vi "Initialize Sweep Waveform.vi"(8 "error in (no error)":errorcluster, 11 "Generator in":refnum<class "Generator.lvclass">) -> (0 "error out":errorcluster, 2 "Waveforms":waveform(dbl)[](array[waveform]), 3 "Generator out":refnum<class "Generator.lvclass">)   [LabVIEW 2019, in "Generator.lvclass"]
uses:
  Generator.lvclass
  Generator.lvclass/Generator.ctl
  <vilib>/Utility/error.llb/Error Cluster From Error Code.vi
  <vilib>/ErrorRing/Error Ring.xnode
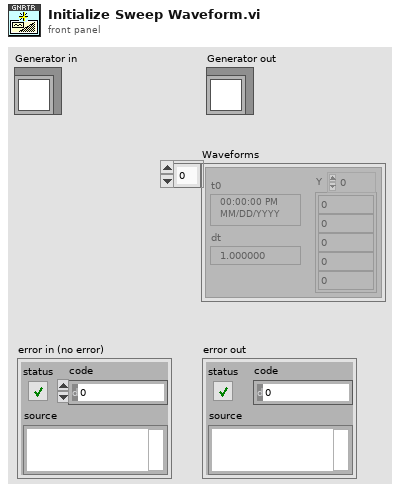
[diagram p1: front panel]
types:
  T1 = typedef "Generator.lvclass/AO.Channel--Cluster--Array.ctl" = T2[]
  T2 = typedef "Generator.lvclass/AO.Channel--Cluster.ctl" = cluster{"Enable?":bool, "Channel":i32, "Amplitude":dbl, "Offset":dbl, "Frequency":dbl, "Phase":dbl, "Function":T3, "Sweeping?":bool, "Limit AC?":bool, "Limit DC?":bool, "Duty Cycle?":bool, "Duty Cycle":dbl}
  T3 = typedef "Generator.lvclass/AO.Channel.Function--Enum.ctl" = enum16{"sine", "square", "triangle", "saw"}
  T4 = typedef "Generator.lvclass/Sweep.Channel--Cluster--Array.ctl" = T5[]
  T5 = typedef "Generator.lvclass/Sweep.Channel--Cluster.ctl" = cluster{"Enable?":bool, "Channel":u16, "Start":dbl, "End":dbl, "Pattern":T6, "Table":dbl[]}
  T6 = typedef "Generator.lvclass/Sweep.Pattern--Enum.ctl" = enum16{"Ramp /", "Ramp /\\", "Smooth Ramp _/", "Smooth Ramp _/\\_", "Table"}
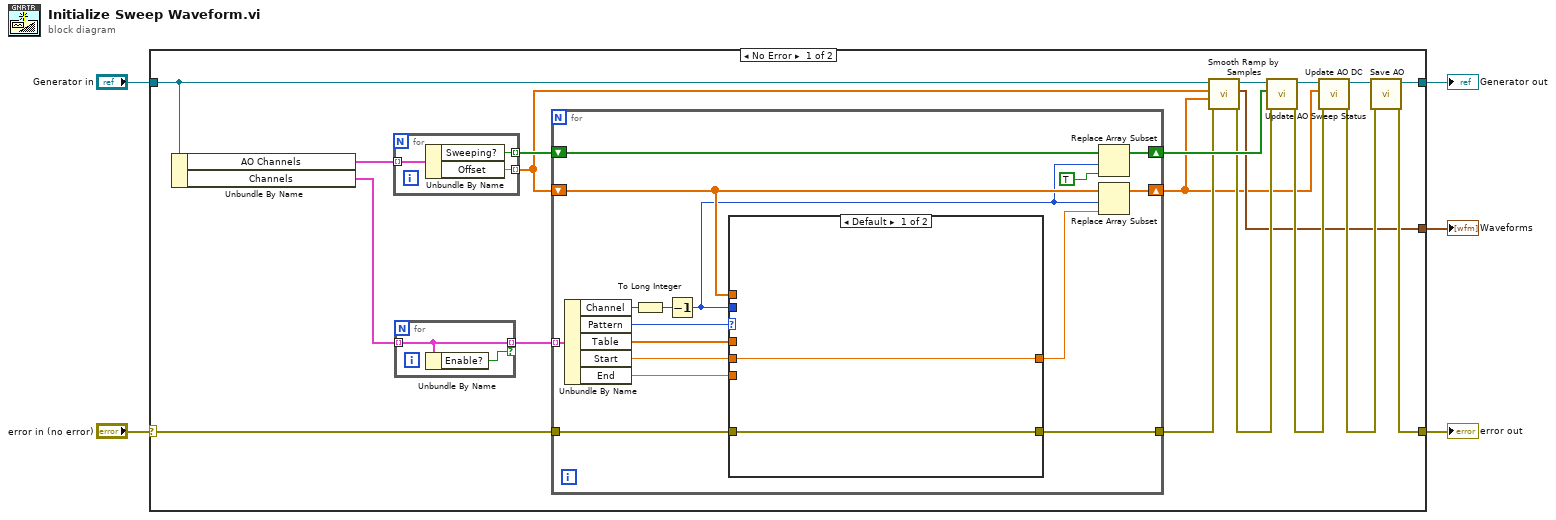
[diagram p0: block diagram]
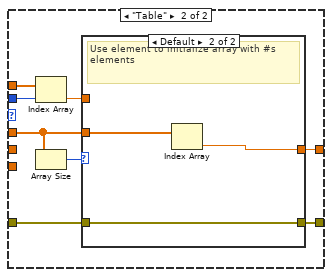
[diagram p2: hidden frame]
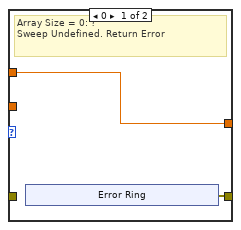
[diagram p3: hidden frame]
diagram:
  n1 = case shown="No Error" "error in (no error)" {
    selector: "error in (no error)" -> [w11 w67]
    tunnel: "Generator in" -> [w12 w66]
    tunnel: [w15 w67] -> w2
    tunnel: [w14 w66] -> w1
    tunnel: [w7 _] -> w3
    frame No Error {
      n2 = Unbundle By Name(w12) -> ("AO Channels"=w22:T1, "Channels"=w21:T4)
      n3 = for {
        tunnel: [w65] -> w8 mode=indexing
        tunnel: [w64] -> w23 mode=indexing
        tunnel: w22 -> [w63] mode=indexing
        n4 = Unbundle By Name(w63) -> ("Sweeping?"=w64:bool, "Offset"=w65:dbl)
      }
      n5 = for {
        tunnel: w21 -> [w62] mode=indexing
        tunnel: [w62] -> w24 mode=indexing if=w61
        n6 = Unbundle By Name(w62) -> ("Enable?"=w61:bool)
      }
      n7 = for {
        tunnel: w11 -> [w40]
        tunnel: w24 -> [w35] mode=indexing
        tunnel: [w34] -> w10
        shift-right: [w30] -> w18
        shift-left: w23 -> [w32]
        shift-right: [w31] -> w6
        shift-left: w8 -> [w29]
        n8 = Unbundle By Name(w35) -> ("Channel"=w28:u16, "Pattern"=w38:T6, "Table"=w39:dbl[], "Start"=w37:dbl, "End"=w36:dbl)
        n9 = To Long Integer(number=w28) -> (32bit integer=w26:i32)
        n10 = Decrement(x=w26) -> (x-1=w25:i32)
        n11 = case shown="Default" w38 {
          tunnel: w36 -> [_ _]
          tunnel: w37 -> [w41 _]
          tunnel: [w42 w49] -> w34
          tunnel: w40 -> [w42 w50]
          tunnel: w39 -> [_ w48]
          tunnel: w29 -> [_ w45]
          tunnel: w25 -> [_ w44]
          tunnel: [w41 w46] -> w27
          frame Default {
          }
          frame "Table" {
            n12 = Index Array(array=w45, index=w44) -> (element=w43:dbl)
            n13 = Array Size(array=w48) -> (size(s)=w47:i32)
            n14 = case shown="Default" w47 {
              tunnel: w50 -> [_ w59]
              tunnel: [w52 w59] -> w49
              tunnel: w48 -> [_ w60]
              tunnel: [w51 w58] -> w46
              tunnel: w43 -> [w51 _]
              frame 0 {
                # "Array Size = 0: ?\nSweep Undefined. Return Error"
                n15 = xnode "Error Ring"() -> ("error out"=w52:errorcluster)
              }
              frame Default {
                # "Use element to initialize array with #s elements"
                n16 = Index Array(array=w60) -> (element=w58:dbl)  [unwired: 1 in]
              }
            }
          }
        }
        n17 = Replace Array Subset(array=w32, new element=TRUE ("new element/subarray"), index=w25) -> (w30:bool[])
        n18 = Replace Array Subset(array=w29, new element=w27, index=w25) -> (w31:dbl[])
      }
      n19 = call "Smooth Ramp by Samples.vi"("error in (no error)"=w10, "End"=w6, "Start"=w8, "Generator in"=w12) -> ("Error out"=w9:errorcluster, "Waveforms out"=w7:waveform(dbl)[], "Generator out"=w13:refnum<class "Generator.lvclass">)  [unwired: 5 in]
      n20 = call "Update AO Sweep Status.vi"("error in (no error)"=w9, "Channels: AO.Sweeping?"=w18, "Generator in"=w13) -> ("error out"=w17:errorcluster, "Generator out"=w19:refnum<class "Generator.lvclass">)  [unwired: 7 in]
      n21 = call "Update AO DC.vi"("error in (no error)"=w17, "AO.DC (V)"=w6, "Generator in"=w19) -> ("error out"=w16:errorcluster, "Generator out"=w20:refnum<class "Generator.lvclass">)  [unwired: 7 in]
      n22 = call "Save AO.vi"("error in (no error)"=w16, "Generator in"=w20) -> ("error out"=w15:errorcluster, "Generator out"=w14:refnum<class "Generator.lvclass">)  [unwired: 8 in]
    }
    frame Error {
    }
  }
  "Generator out" <- w1
  "error out" <- w2
  "Waveforms" <- w3
